vi "ABCtoAlphaBeta_3PhaseUnitaryMagnitude_src.vi"(0 "A":sgl, 5 "B":sgl, 7 "C":sgl) -> (4 "alpha":sgl, 6 "beta":sgl)   [LabVIEW 2015]
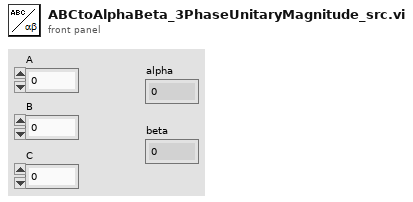
[diagram p1: front panel]
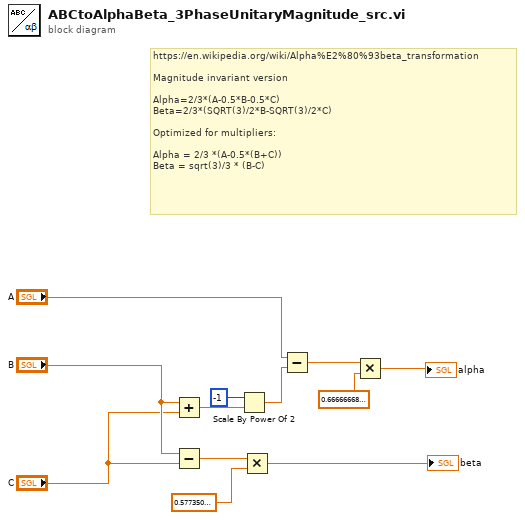
[diagram p0: block diagram]
diagram:
  # "https://en.wikipedia.org/wiki/Alpha%E2%80%93beta_transformation\n\nMagnitude invariant version\n\nAlpha=2/3*(A-0.5*B-0.5*C)\nBeta=2/3*(SQRT(3)/2*B-SQRT(3)/2*C)\n\nOptimized for multipliers:\n\nAlpha = 2/3 *(A-0.5*(B+C))\nBeta = sqrt(3)/3 * (B-C)"
  n1 = Add(x="B", y="C") -> (x+y=w5:sgl)
  n2 = Subtract(x="B", y="C") -> (x-y=w7:sgl)
  n3 = Scale By Power Of 2(n=i16 -1, x=w5) -> (x*2^n=w3:sgl)
  n4 = Multiply(x=w7, y=sgl 0.57735) -> (x*y=→"beta":sgl)
  n5 = Subtract(x="A", y=w3) -> (x-y=w2:sgl)
  n6 = Multiply(x=w2, y=sgl 0.6666667) -> (x*y=→"alpha":sgl)
